vi "Begin.vi"(8 "error in":errorcluster) -> (0 "error out":errorcluster)   [LabVIEW 2017]
doc: "Called before other user functions, this VI is expected to open initial I/O refnums, load in file data, and do all program initialization. Notice that the <B>error out</B> terminal is simply used for data flow. Wiring it to other structures or subVIs ensures that this VI runs first."
uses:
  <vilib>/Rock Robotics/WPI/DriverStation/WPI_DriverStationRobotMode2.ctl
  <vilib>/Rock Robotics/WPI/Joystick/WPI_JoystickDeviceEnum.ctl
  <vilib>/Rock Robotics/WPI/ThirdParty/Phoenix-LabVIEW/Motor Controller/Controls/CTRE_Phoenix_MotorControl_FeedbackDevice.ctl
  <vilib>/Rock Robotics/WPI/ThirdParty/Phoenix-LabVIEW/Motor Controller/Controls/CTRE_Phoenix_MotorControl_NeutralMode.ctl
  <vilib>/Rock Robotics/WPI/ThirdParty/Phoenix-LabVIEW/Motor Controller/Controls/CTRE_Phoenix_MotorControl_ControlMode.ctl
  Robot Global Data.vi
  <vilib>/Rock Robotics/WPI/ThirdParty/Phoenix-LabVIEW/Pigeon IMU/CTRE_PigeonIMU_Open_CAN.vi
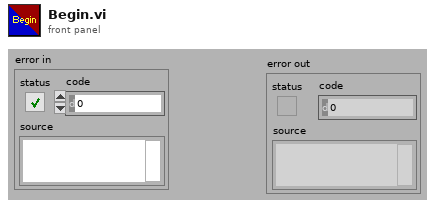
[diagram p1: front panel]
types:
  T1 = typedef "CTRE_Phoenix_MotorControl_ControlMode.ctl" = u16
  T2 = typedef "CTRE_Phoenix_MotorControl_NeutralMode.ctl" = enum8{"EEPROMSetting", "Override to Coast", "Override to Brake"}
  T3 = typedef "CTRE_Phoenix_MotorControl_FeedbackDevice.ctl" = i8
  T4 = typedef "WPI_JoystickDeviceEnum.ctl" = enum16{"USB 0", "USB 1", "USB 2", "USB 3", "USB 4", "USB 5"}
  T5 = typedef "WPI_DriverStationRobotMode2.ctl" = enum16{"Autonomous Disabled", "Autonomous Enabled", "Teleop Disabled", "Teleop Enabled", "Disconnected", "Finish", "Test Disabled", "Test Enabled", "Emergency Stopped"}
  T6 = typedef "CTRE_PigeonIMU_DeviceRef.ctl" = cluster{"DeviceStatus":errorcluster, "Device Number":u8, "Type":T7, "Device ID":u32, "Handle":u64, "UsageFrame":u32, "Library Path":path}
  T7 = typedef "CTRE_PigeonIMU_ConnectionType.ctl" = u32
  T8 = typedef "WPI_JoystickDevRef.ctl" = cluster{"Device":T4}
  T9 = typedef "WPI_MotorControlDeviceRef.ctl" = cluster{"DeviceStatus":errorcluster, "Type":T10, "PWM":cluster{"PWM Channel":T11, "DeadBand":T12}, "CAN":cluster{"Device Number":u8, "SetOutput VI Ref":variant, "GetOutput VI Ref":variant, "Enable VI Ref":variant, "Disable VI Ref":variant, "Data":variant}, "Invert":bool, "DIO PWM":cluster{"PWM \"Enable\" Channel":T11, "DIOChannel":T13, "PWM Rate":dbl}}
  T10 = typedef "WPI_MotorControlType.ctl" = enum16{"PWM", "CAN", "DIO PWM"}
  T11 = typedef "FPGA_DIOPWMChannel.ctl" = enum8{"PWM 0", "PWM 1", "PWM 2", "PWM 3", "PWM 4", "PWM 5", "PWM 6", "PWM 7", "PWM 8", "PWM 9", "PWM MXP 0", "PWM MXP 1", "PWM MXP 2", "PWM MXP 3", "PWM MXP 4", "PWM MXP 5", "PWM MXP 6", "PWM MXP 7", "PWM MXP 8", "PWM MXP 9", "Invalid"}
  T12 = typedef "WPI_PWMDeadband.ctl" = cluster{"Name":string, "maxPositivePwm":i32, "minPositivePwm":i32, "centerPwm":i32, "maxNegativePwm":i32, "minNegativePwm":i32, "angularRange":u16}
  T13 = typedef "FPGA_DIOChannel.ctl" = enum8{"DIO 0", "DIO 1", "DIO 2", "DIO 3", "DIO 4", "DIO 5", "DIO 6", "DIO 7", "DIO 8", "DIO 9", "DIO MXP 0", "DIO MXP 1", "DIO MXP 2", "DIO MXP 3", "DIO MXP 4", "DIO MXP 5", "DIO MXP 6", "DIO MXP 7", "DIO MXP 8", "DIO MXP 9", "DIO MXP 10", "DIO MXP 11", "DIO MXP 12", "DIO MXP 13", "DIO MXP 14", "DIO MXP 15", "SPI Port CS1", "SPI Port CS2", "SPI Port CS3", "SPI Port MISO", "SPI Port MOSI", "Invalid"}
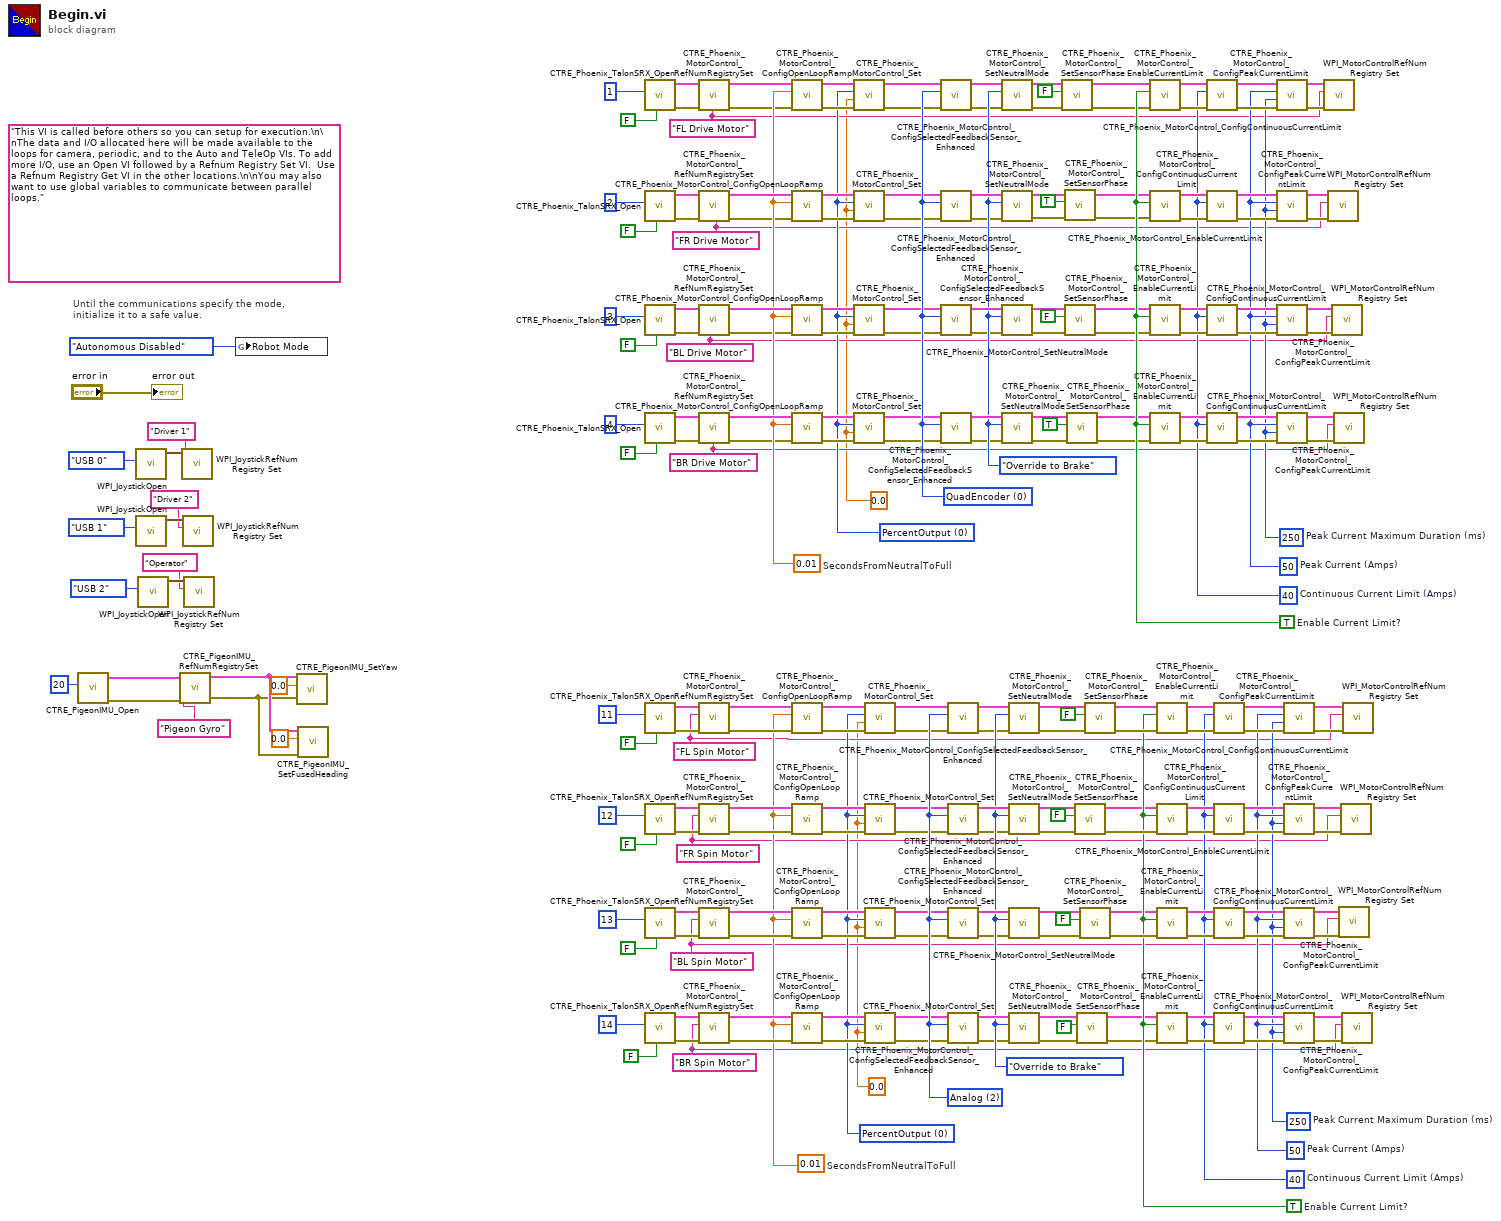
[diagram p0: block diagram]
diagram:
  w1 = 0.0 ("Output")
  w2 = 0.0 ("Output")
  w11 = T1 0 items=["PercentOutput"=0, "Position"=1, "Velocity"=2, "Current"=3, "Follower"=5, "MotionProfile"=6, "MotionMagic"=7, "MotionMagicArc"=8, "MotionProfileArc"=10, "Disabled"=15] ("Control Mode")
  w16 = T1 0 items=["PercentOutput"=0, "Position"=1, "Velocity"=2, "Current"=3, "Follower"=5, "MotionProfile"=6, "MotionMagic"=7, "MotionMagicArc"=8, "MotionProfileArc"=10, "Disabled"=15] ("Control Mode")
  w37 = 0.01  # SecondsFromNeutralToFull
  w94 = CTRE_Phoenix_MotorControl_NeutralMode."Override to Brake" ("Motor Control Neutral Mode")
  w95 = T3 0 items=["None"=-1, "QuadEncoder"=0, "Analog"=2, "Tachometer"=4, "Pulse Width Encoded Position"=8, "Sensor Sum (S0 + S1)"=9, "Sensor Difference (D0 - D1)"=10, "Remote Source 0"=11, "Remote Source 1"=12, "Software Emulated"=15] ("Feedback Device")
  w96 = 0.01  # SecondsFromNeutralToFull
  w7 = "BR Drive Motor" ("refnum name")
  w8 = "BL Drive Motor" ("refnum name")
  w9 = "FR Drive Motor" ("refnum name")
  w62 = 250  # Peak Current Maximum Duration (ms)
  w63 = 50  # Peak Current (Amps)
  w65 = 40  # Continuous Current Limit (Amps)
  w64 = TRUE  # Enable Current Limit?
  w10 = "FL Drive Motor" ("refnum name")
  w173 = CTRE_Phoenix_MotorControl_NeutralMode."Override to Brake" ("Motor Control Neutral Mode")
  w174 = T3 2 items=["None"=-1, "QuadEncoder"=0, "Analog"=2, "Tachometer"=4, "Pulse Width Encoded Position"=8, "Sensor Sum (S0 + S1)"=9, "Sensor Difference (D0 - D1)"=10, "Remote Source 0"=11, "Remote Source 1"=12, "Software Emulated"=15] ("Feedback Device")
  w3 = "BR Spin Motor" ("refnum name")
  w4 = "BL Spin Motor" ("refnum name")
  w5 = "FR Spin Motor" ("refnum name")
  w138 = 250  # Peak Current Maximum Duration (ms)
  w139 = 50  # Peak Current (Amps)
  w141 = 40  # Continuous Current Limit (Amps)
  w140 = TRUE  # Enable Current Limit?
  w6 = "FL Spin Motor" ("refnum name")
  (unwired) "This VI is called before others so you can setup for execution.\n\nThe data and I/O allocated here will be made available to the loops for camera, periodic, and to the Auto and TeleOp VIs. To add more I/O, use an Open VI followed by a Refnum Registry Set VI.  Use a Refnum Registry Get VI in the other locations.\n\nYou may also want to use global variables to communicate between parallel loops."
  # "Until the communications specify the mode,\ninitialize it to a safe value."
  n1 = call-poly <vilib>:"CTRE_PigeonIMU_Open.vi"("Device Number"=u8 20) -> ("error out"=w206:errorcluster, "PigeonIMUDevRef"=w205:T6)  [unwired: 9 in]
  n2 = call <vilib>:"WPI_JoystickOpen.vi"("JoystickDevice"=WPI_JoystickDeviceEnum."USB 0") -> ("JoystickDevRef"=w215:T8)  [unwired: 10 in]
  n3 = call <vilib>:"WPI_JoystickOpen.vi"("JoystickDevice"=WPI_JoystickDeviceEnum."USB 1") -> ("JoystickDevRef"=w214:T8)  [unwired: 10 in]
  n4 = call <vilib>:"WPI_JoystickOpen.vi"("JoystickDevice"=WPI_JoystickDeviceEnum."USB 2") -> ("JoystickDevRef"=w213:T8)  [unwired: 10 in]
  n5 = call <vilib>:"CTRE_PigeonIMU_RefNumRegistrySet.vi"("error in (no error)"=w206, "refnum name"="Pigeon Gyro", "PigeonIMUDevRef"=w205) -> ("error out"=w201:errorcluster, "PigeonIMUDevRef"=w202:T6)  [unwired: 7 in]
  n6 = call <vilib>:"WPI_JoystickRefNum Registry Set.vi"("refnum name"="Driver 1", "JoystickDevRef"=w215) -> ()  [unwired: 8 in, 2 out]
  n7 = call <vilib>:"WPI_JoystickRefNum Registry Set.vi"("refnum name"="Driver 2", "JoystickDevRef"=w214) -> ()  [unwired: 8 in, 2 out]
  n8 = call <vilib>:"WPI_JoystickRefNum Registry Set.vi"("refnum name"="Operator", "JoystickDevRef"=w213) -> ()  [unwired: 8 in, 2 out]
  n9 = global write "Robot Global Data.vi" "Robot Mode"(WPI_DriverStationRobotMode2."Autonomous Disabled" ("Robot Mode")) -> ()
  n10 = call <vilib>:"CTRE_PigeonIMU_SetYaw.vi"("error in (no error)"=w201, "Value"=0.0, "PigeonIMUDevRef"=w202) -> ()  [unwired: 7 in, 2 out]
  n11 = call <vilib>:"CTRE_PigeonIMU_SetFusedHeading.vi"("error in (no error)"=w201, "Value"=0.0, "PigeonIMUDevRef 2"=w202) -> ()  [unwired: 7 in, 2 out]
  n12 = call <vilib>:"CTRE_Phoenix_TalonSRX_Open.vi"("Invert"=FALSE, "Device Number"=u8 1) -> ("error out"=w93:errorcluster, "CAN Talon SRX Ref"=w119:T9)  [unwired: 8 in]
  n13 = call <vilib>:"CTRE_Phoenix_TalonSRX_Open.vi"("Invert"=FALSE, "Device Number"=u8 2) -> ("error out"=w89:errorcluster, "CAN Talon SRX Ref"=w110:T9)  [unwired: 8 in]
  n14 = call <vilib>:"CTRE_Phoenix_TalonSRX_Open.vi"("Invert"=FALSE, "Device Number"=u8 3) -> ("error out"=w85:errorcluster, "CAN Talon SRX Ref"=w105:T9)  [unwired: 8 in]
  n15 = call <vilib>:"CTRE_Phoenix_TalonSRX_Open.vi"("Invert"=FALSE, "Device Number"=u8 4) -> ("error out"=w81:errorcluster, "CAN Talon SRX Ref"=w100:T9)  [unwired: 8 in]
  n16 = call <vilib>:"CTRE_Phoenix_TalonSRX_Open.vi"("Invert"=FALSE, "Device Number"=u8 11) -> ("error out"=w172:errorcluster, "CAN Talon SRX Ref"=w197:T9)  [unwired: 8 in]
  n17 = call <vilib>:"CTRE_Phoenix_TalonSRX_Open.vi"("Invert"=FALSE, "Device Number"=u8 12) -> ("error out"=w168:errorcluster, "CAN Talon SRX Ref"=w188:T9)  [unwired: 8 in]
  n18 = call <vilib>:"CTRE_Phoenix_TalonSRX_Open.vi"("Invert"=FALSE, "Device Number"=u8 13) -> ("error out"=w164:errorcluster, "CAN Talon SRX Ref"=w183:T9)  [unwired: 8 in]
  n19 = call <vilib>:"CTRE_Phoenix_TalonSRX_Open.vi"("Invert"=FALSE, "Device Number"=u8 14) -> ("error out"=w160:errorcluster, "CAN Talon SRX Ref"=w178:T9)  [unwired: 8 in]
  n20 = call <vilib>:"CTRE_Phoenix_MotorControl_RefNumRegistrySet.vi"("error in (no error)"=w93, "refnum name"=w10, "PhoenixMotorControlDevRef"=w119) -> ("error out"=w92:errorcluster, "PhoenixMotorControlDevRef"=w114:T9)  [unwired: 7 in]
  n21 = call <vilib>:"CTRE_Phoenix_MotorControl_RefNumRegistrySet.vi"("error in (no error)"=w89, "refnum name"=w9, "PhoenixMotorControlDevRef"=w110) -> ("error out"=w88:errorcluster, "PhoenixMotorControlDevRef"=w109:T9)  [unwired: 7 in]
  n22 = call <vilib>:"CTRE_Phoenix_MotorControl_RefNumRegistrySet.vi"("error in (no error)"=w85, "refnum name"=w8, "PhoenixMotorControlDevRef"=w105) -> ("error out"=w84:errorcluster, "PhoenixMotorControlDevRef"=w104:T9)  [unwired: 7 in]
  n23 = call <vilib>:"CTRE_Phoenix_MotorControl_RefNumRegistrySet.vi"("error in (no error)"=w81, "refnum name"=w7, "PhoenixMotorControlDevRef"=w100) -> ("error out"=w80:errorcluster, "PhoenixMotorControlDevRef"=w99:T9)  [unwired: 7 in]
  n24 = call <vilib>:"CTRE_Phoenix_MotorControl_RefNumRegistrySet.vi"("error in (no error)"=w172, "refnum name"=w6, "PhoenixMotorControlDevRef"=w197) -> ("error out"=w171:errorcluster, "PhoenixMotorControlDevRef"=w192:T9)  [unwired: 7 in]
  n25 = call <vilib>:"CTRE_Phoenix_MotorControl_RefNumRegistrySet.vi"("error in (no error)"=w168, "refnum name"=w5, "PhoenixMotorControlDevRef"=w188) -> ("error out"=w167:errorcluster, "PhoenixMotorControlDevRef"=w187:T9)  [unwired: 7 in]
  n26 = call <vilib>:"CTRE_Phoenix_MotorControl_RefNumRegistrySet.vi"("error in (no error)"=w164, "refnum name"=w4, "PhoenixMotorControlDevRef"=w183) -> ("error out"=w163:errorcluster, "PhoenixMotorControlDevRef"=w182:T9)  [unwired: 7 in]
  n27 = call <vilib>:"CTRE_Phoenix_MotorControl_RefNumRegistrySet.vi"("error in (no error)"=w160, "refnum name"=w3, "PhoenixMotorControlDevRef"=w178) -> ("error out"=w159:errorcluster, "PhoenixMotorControlDevRef"=w177:T9)  [unwired: 7 in]
  n28 = call <vilib>:"CTRE_Phoenix_MotorControl_ConfigOpenLoopRamp.vi"("error in (no error)"=w92, "secondsFromNeutralToFull"=w96, "PhoenixMotorControlDevRef"=w114) -> ("error out"=w91:errorcluster, "PhoenixMotorControlDevRef"=w113:T9)  [unwired: 7 in]
  n29 = call <vilib>:"CTRE_Phoenix_MotorControl_ConfigOpenLoopRamp.vi"("error in (no error)"=w88, "secondsFromNeutralToFull"=w96, "PhoenixMotorControlDevRef"=w109) -> ("error out"=w87:errorcluster, "PhoenixMotorControlDevRef"=w108:T9)  [unwired: 7 in]
  n30 = call <vilib>:"CTRE_Phoenix_MotorControl_ConfigOpenLoopRamp.vi"("error in (no error)"=w84, "secondsFromNeutralToFull"=w96, "PhoenixMotorControlDevRef"=w104) -> ("error out"=w83:errorcluster, "PhoenixMotorControlDevRef"=w103:T9)  [unwired: 7 in]
  n31 = call <vilib>:"CTRE_Phoenix_MotorControl_ConfigOpenLoopRamp.vi"("error in (no error)"=w80, "secondsFromNeutralToFull"=w96, "PhoenixMotorControlDevRef"=w99) -> ("error out"=w79:errorcluster, "PhoenixMotorControlDevRef"=w98:T9)  [unwired: 7 in]
  n32 = call <vilib>:"CTRE_Phoenix_MotorControl_ConfigOpenLoopRamp.vi"("error in (no error)"=w171, "secondsFromNeutralToFull"=w37, "PhoenixMotorControlDevRef"=w192) -> ("error out"=w170:errorcluster, "PhoenixMotorControlDevRef"=w191:T9)  [unwired: 7 in]
  n33 = call <vilib>:"CTRE_Phoenix_MotorControl_ConfigOpenLoopRamp.vi"("error in (no error)"=w167, "secondsFromNeutralToFull"=w37, "PhoenixMotorControlDevRef"=w187) -> ("error out"=w166:errorcluster, "PhoenixMotorControlDevRef"=w186:T9)  [unwired: 7 in]
  n34 = call <vilib>:"CTRE_Phoenix_MotorControl_ConfigOpenLoopRamp.vi"("error in (no error)"=w163, "secondsFromNeutralToFull"=w37, "PhoenixMotorControlDevRef"=w182) -> ("error out"=w162:errorcluster, "PhoenixMotorControlDevRef"=w181:T9)  [unwired: 7 in]
  n35 = call <vilib>:"CTRE_Phoenix_MotorControl_ConfigOpenLoopRamp.vi"("error in (no error)"=w159, "secondsFromNeutralToFull"=w37, "PhoenixMotorControlDevRef"=w177) -> ("error out"=w158:errorcluster, "PhoenixMotorControlDevRef"=w176:T9)  [unwired: 7 in]
  n36 = call <vilib>:"CTRE_Phoenix_MotorControl_Set.vi"("Output"=w2, "Control Mode"=w11, "PhoenixMotorControlDevRef"=w113) -> ("PhoenixMotorControlDevRef"=w15:T9)  [unwired: 7 in, 1 out]
  n37 = call <vilib>:"CTRE_Phoenix_MotorControl_Set.vi"("Output"=w2, "Control Mode"=w11, "PhoenixMotorControlDevRef"=w108) -> ("PhoenixMotorControlDevRef"=w14:T9)  [unwired: 7 in, 1 out]
  n38 = call <vilib>:"CTRE_Phoenix_MotorControl_Set.vi"("Output"=w2, "Control Mode"=w11, "PhoenixMotorControlDevRef"=w103) -> ("PhoenixMotorControlDevRef"=w13:T9)  [unwired: 7 in, 1 out]
  n39 = call <vilib>:"CTRE_Phoenix_MotorControl_Set.vi"("Output"=w2, "Control Mode"=w11, "PhoenixMotorControlDevRef"=w98) -> ("PhoenixMotorControlDevRef"=w12:T9)  [unwired: 7 in, 1 out]
  n40 = call <vilib>:"CTRE_Phoenix_MotorControl_Set.vi"("Output"=w1, "Control Mode"=w16, "PhoenixMotorControlDevRef"=w191) -> ("PhoenixMotorControlDevRef"=w20:T9)  [unwired: 7 in, 1 out]
  n41 = call <vilib>:"CTRE_Phoenix_MotorControl_Set.vi"("Output"=w1, "Control Mode"=w16, "PhoenixMotorControlDevRef"=w186) -> ("PhoenixMotorControlDevRef"=w19:T9)  [unwired: 7 in, 1 out]
  n42 = call <vilib>:"CTRE_Phoenix_MotorControl_Set.vi"("Output"=w1, "Control Mode"=w16, "PhoenixMotorControlDevRef"=w181) -> ("PhoenixMotorControlDevRef"=w18:T9)  [unwired: 7 in, 1 out]
  n43 = call <vilib>:"CTRE_Phoenix_MotorControl_Set.vi"("Output"=w1, "Control Mode"=w16, "PhoenixMotorControlDevRef"=w176) -> ("PhoenixMotorControlDevRef"=w17:T9)  [unwired: 7 in, 1 out]
  n44 = call <vilib>:"CTRE_Phoenix_MotorControl_ConfigSelectedFeedbackSensor_Enhanced.vi"("error in (no error)"=w91, "Feedback Device"=w95, "PhoenixMotorControlDevRef"=w15) -> ("error out"=w90:errorcluster, "PhoenixMotorControlDevRef"=w112:T9)  [unwired: 7 in]
  n45 = call <vilib>:"CTRE_Phoenix_MotorControl_ConfigSelectedFeedbackSensor_Enhanced.vi"("error in (no error)"=w87, "Feedback Device"=w95, "PhoenixMotorControlDevRef"=w14) -> ("error out"=w86:errorcluster, "PhoenixMotorControlDevRef"=w107:T9)  [unwired: 7 in]
  n46 = call <vilib>:"CTRE_Phoenix_MotorControl_ConfigSelectedFeedbackSensor_Enhanced.vi"("error in (no error)"=w83, "Feedback Device"=w95, "PhoenixMotorControlDevRef"=w13) -> ("error out"=w82:errorcluster, "PhoenixMotorControlDevRef"=w102:T9)  [unwired: 7 in]
  n47 = call <vilib>:"CTRE_Phoenix_MotorControl_ConfigSelectedFeedbackSensor_Enhanced.vi"("error in (no error)"=w79, "Feedback Device"=w95, "PhoenixMotorControlDevRef"=w12) -> ("error out"=w78:errorcluster, "PhoenixMotorControlDevRef"=w97:T9)  [unwired: 7 in]
  n48 = call <vilib>:"CTRE_Phoenix_MotorControl_ConfigSelectedFeedbackSensor_Enhanced.vi"("error in (no error)"=w170, "Feedback Device"=w174, "PhoenixMotorControlDevRef"=w20) -> ("error out"=w169:errorcluster, "PhoenixMotorControlDevRef"=w190:T9)  [unwired: 7 in]
  n49 = call <vilib>:"CTRE_Phoenix_MotorControl_ConfigSelectedFeedbackSensor_Enhanced.vi"("error in (no error)"=w166, "Feedback Device"=w174, "PhoenixMotorControlDevRef"=w19) -> ("error out"=w165:errorcluster, "PhoenixMotorControlDevRef"=w185:T9)  [unwired: 7 in]
  n50 = call <vilib>:"CTRE_Phoenix_MotorControl_ConfigSelectedFeedbackSensor_Enhanced.vi"("error in (no error)"=w162, "Feedback Device"=w174, "PhoenixMotorControlDevRef"=w18) -> ("error out"=w161:errorcluster, "PhoenixMotorControlDevRef"=w180:T9)  [unwired: 7 in]
  n51 = call <vilib>:"CTRE_Phoenix_MotorControl_ConfigSelectedFeedbackSensor_Enhanced.vi"("error in (no error)"=w158, "Feedback Device"=w174, "PhoenixMotorControlDevRef"=w17) -> ("error out"=w157:errorcluster, "PhoenixMotorControlDevRef"=w175:T9)  [unwired: 7 in]
  n52 = call <vilib>:"CTRE_Phoenix_MotorControl_SetNeutralMode.vi"("error in (no error)"=w90, "Motor Control Neutral Mode"=w94, "PhoenixMotorControlDevRef"=w112) -> ("error out"=w51:errorcluster, "PhoenixMotorControlDevRef"=w52:T9)  [unwired: 7 in]
  n53 = call <vilib>:"CTRE_Phoenix_MotorControl_SetNeutralMode.vi"("error in (no error)"=w86, "Motor Control Neutral Mode"=w94, "PhoenixMotorControlDevRef"=w107) -> ("error out"=w47:errorcluster, "PhoenixMotorControlDevRef"=w48:T9)  [unwired: 7 in]
  n54 = call <vilib>:"CTRE_Phoenix_MotorControl_SetNeutralMode.vi"("error in (no error)"=w82, "Motor Control Neutral Mode"=w94, "PhoenixMotorControlDevRef"=w102) -> ("error out"=w41:errorcluster, "PhoenixMotorControlDevRef"=w42:T9)  [unwired: 7 in]
  n55 = call <vilib>:"CTRE_Phoenix_MotorControl_SetNeutralMode.vi"("error in (no error)"=w78, "Motor Control Neutral Mode"=w94, "PhoenixMotorControlDevRef"=w97) -> ("error out"=w56:errorcluster, "PhoenixMotorControlDevRef"=w57:T9)  [unwired: 7 in]
  n56 = call <vilib>:"CTRE_Phoenix_MotorControl_SetNeutralMode.vi"("error in (no error)"=w169, "Motor Control Neutral Mode"=w173, "PhoenixMotorControlDevRef"=w190) -> ("error out"=w152:errorcluster, "PhoenixMotorControlDevRef"=w133:T9)  [unwired: 7 in]
  n57 = call <vilib>:"CTRE_Phoenix_MotorControl_SetNeutralMode.vi"("error in (no error)"=w165, "Motor Control Neutral Mode"=w173, "PhoenixMotorControlDevRef"=w185) -> ("error out"=w149:errorcluster, "PhoenixMotorControlDevRef"=w132:T9)  [unwired: 7 in]
  n58 = call <vilib>:"CTRE_Phoenix_MotorControl_SetNeutralMode.vi"("error in (no error)"=w161, "Motor Control Neutral Mode"=w173, "PhoenixMotorControlDevRef"=w180) -> ("error out"=w146:errorcluster, "PhoenixMotorControlDevRef"=w131:T9)  [unwired: 7 in]
  n59 = call <vilib>:"CTRE_Phoenix_MotorControl_SetNeutralMode.vi"("error in (no error)"=w157, "Motor Control Neutral Mode"=w173, "PhoenixMotorControlDevRef"=w175) -> ("error out"=w129:errorcluster, "PhoenixMotorControlDevRef"=w130:T9)  [unwired: 7 in]
  n60 = call <vilib>:"CTRE_Phoenix_MotorControl_SetSensorPhase.vi"("error in (no error)"=w51, "PhaseSensor"=FALSE, "PhoenixMotorControlDevRef"=w52) -> ("error out"=w49:errorcluster, "PhoenixMotorControlDevRef"=w50:T9)  [unwired: 7 in]
  n61 = call <vilib>:"CTRE_Phoenix_MotorControl_SetSensorPhase.vi"("error in (no error)"=w47, "PhaseSensor"=TRUE, "PhoenixMotorControlDevRef"=w48) -> ("error out"=w46:errorcluster, "PhoenixMotorControlDevRef"=w45:T9)  [unwired: 7 in]
  n62 = call <vilib>:"CTRE_Phoenix_MotorControl_SetSensorPhase.vi"("error in (no error)"=w41, "PhaseSensor"=FALSE, "PhoenixMotorControlDevRef"=w42) -> ("error out"=w40:errorcluster, "PhoenixMotorControlDevRef"=w39:T9)  [unwired: 7 in]
  n63 = call <vilib>:"CTRE_Phoenix_MotorControl_SetSensorPhase.vi"("error in (no error)"=w56, "PhaseSensor"=TRUE ("Invert?"), "PhoenixMotorControlDevRef"=w57) -> ("error out"=w54:errorcluster, "PhoenixMotorControlDevRef"=w53:T9)  [unwired: 7 in]
  n64 = call <vilib>:"CTRE_Phoenix_MotorControl_SetSensorPhase.vi"("PhaseSensor"=FALSE, "PhoenixMotorControlDevRef"=w132) -> ("PhoenixMotorControlDevRef"=w124:T9)  [unwired: 8 in, 1 out]
  n65 = call <vilib>:"CTRE_Phoenix_MotorControl_SetSensorPhase.vi"("PhaseSensor"=FALSE, "PhoenixMotorControlDevRef"=w130) -> ("PhoenixMotorControlDevRef"=w128:T9)  [unwired: 8 in, 1 out]
  n66 = call <vilib>:"CTRE_Phoenix_MotorControl_SetSensorPhase.vi"("PhaseSensor"=FALSE, "PhoenixMotorControlDevRef"=w131) -> ("PhoenixMotorControlDevRef"=w126:T9)  [unwired: 8 in, 1 out]
  n67 = call <vilib>:"CTRE_Phoenix_MotorControl_SetSensorPhase.vi"("PhaseSensor"=FALSE, "PhoenixMotorControlDevRef"=w133) -> ("PhoenixMotorControlDevRef"=w122:T9)  [unwired: 8 in, 1 out]
  n68 = call <vilib>:"CTRE_Phoenix_MotorControl_EnableCurrentLimit.vi"("error in (no error)"=w49, "Enable Current Limit?"=w64, "PhoenixMotorControlDevRef"=w50) -> ("error out"=w73:errorcluster, "PhoenixMotorControlDevRef"=w75:T9)  [unwired: 7 in]
  n69 = call <vilib>:"CTRE_Phoenix_MotorControl_EnableCurrentLimit.vi"("error in (no error)"=w46, "Enable Current Limit?"=w64, "PhoenixMotorControlDevRef"=w45) -> ("error out"=w71:errorcluster, "PhoenixMotorControlDevRef"=w77:T9)  [unwired: 7 in]
  n70 = call <vilib>:"CTRE_Phoenix_MotorControl_EnableCurrentLimit.vi"("error in (no error)"=w40, "Enable Current Limit?"=w64, "PhoenixMotorControlDevRef"=w39) -> ("error out"=w69:errorcluster, "PhoenixMotorControlDevRef"=w118:T9)  [unwired: 7 in]
  n71 = call <vilib>:"CTRE_Phoenix_MotorControl_EnableCurrentLimit.vi"("error in (no error)"=w54, "Enable Current Limit?"=w64, "PhoenixMotorControlDevRef"=w53) -> ("error out"=w67:errorcluster, "PhoenixMotorControlDevRef"=w116:T9)  [unwired: 7 in]
  n72 = call <vilib>:"CTRE_Phoenix_MotorControl_EnableCurrentLimit.vi"("error in (no error)"=w152, "Enable Current Limit?"=w140, "PhoenixMotorControlDevRef"=w122) -> ("error out"=w151:errorcluster, "PhoenixMotorControlDevRef"=w154:T9)  [unwired: 7 in]
  n73 = call <vilib>:"CTRE_Phoenix_MotorControl_EnableCurrentLimit.vi"("error in (no error)"=w149, "Enable Current Limit?"=w140, "PhoenixMotorControlDevRef"=w124) -> ("error out"=w148:errorcluster, "PhoenixMotorControlDevRef"=w156:T9)  [unwired: 7 in]
  n74 = call <vilib>:"CTRE_Phoenix_MotorControl_EnableCurrentLimit.vi"("error in (no error)"=w146, "Enable Current Limit?"=w140, "PhoenixMotorControlDevRef"=w126) -> ("error out"=w145:errorcluster, "PhoenixMotorControlDevRef"=w196:T9)  [unwired: 7 in]
  n75 = call <vilib>:"CTRE_Phoenix_MotorControl_EnableCurrentLimit.vi"("error in (no error)"=w129, "Enable Current Limit?"=w140, "PhoenixMotorControlDevRef"=w128) -> ("error out"=w143:errorcluster, "PhoenixMotorControlDevRef"=w194:T9)  [unwired: 7 in]
  n76 = call <vilib>:"CTRE_Phoenix_MotorControl_ConfigContinuousCurrentLimit.vi"("error in (no error)"=w73, "Continuous Current Limit (Amps)"=w65, "PhoenixMotorControlDevRef"=w75) -> ("error out"=w72:errorcluster, "PhoenixMotorControlDevRef"=w74:T9)  [unwired: 7 in]
  n77 = call <vilib>:"CTRE_Phoenix_MotorControl_ConfigContinuousCurrentLimit.vi"("error in (no error)"=w71, "Continuous Current Limit (Amps)"=w65, "PhoenixMotorControlDevRef"=w77) -> ("error out"=w70:errorcluster, "PhoenixMotorControlDevRef"=w76:T9)  [unwired: 7 in]
  n78 = call <vilib>:"CTRE_Phoenix_MotorControl_ConfigContinuousCurrentLimit.vi"("error in (no error)"=w69, "Continuous Current Limit (Amps)"=w65, "PhoenixMotorControlDevRef"=w118) -> ("error out"=w68:errorcluster, "PhoenixMotorControlDevRef"=w117:T9)  [unwired: 7 in]
  n79 = call <vilib>:"CTRE_Phoenix_MotorControl_ConfigContinuousCurrentLimit.vi"("error in (no error)"=w67, "Continuous Current Limit (Amps)"=w65, "PhoenixMotorControlDevRef"=w116) -> ("error out"=w66:errorcluster, "PhoenixMotorControlDevRef"=w115:T9)  [unwired: 7 in]
  n80 = call <vilib>:"CTRE_Phoenix_MotorControl_ConfigContinuousCurrentLimit.vi"("error in (no error)"=w151, "Continuous Current Limit (Amps)"=w141, "PhoenixMotorControlDevRef"=w154) -> ("error out"=w150:errorcluster, "PhoenixMotorControlDevRef"=w153:T9)  [unwired: 7 in]
  n81 = call <vilib>:"CTRE_Phoenix_MotorControl_ConfigContinuousCurrentLimit.vi"("error in (no error)"=w148, "Continuous Current Limit (Amps)"=w141, "PhoenixMotorControlDevRef"=w156) -> ("error out"=w147:errorcluster, "PhoenixMotorControlDevRef"=w155:T9)  [unwired: 7 in]
  n82 = call <vilib>:"CTRE_Phoenix_MotorControl_ConfigContinuousCurrentLimit.vi"("error in (no error)"=w145, "Continuous Current Limit (Amps)"=w141, "PhoenixMotorControlDevRef"=w196) -> ("error out"=w144:errorcluster, "PhoenixMotorControlDevRef"=w195:T9)  [unwired: 7 in]
  n83 = call <vilib>:"CTRE_Phoenix_MotorControl_ConfigContinuousCurrentLimit.vi"("error in (no error)"=w143, "Continuous Current Limit (Amps)"=w141, "PhoenixMotorControlDevRef"=w194) -> ("error out"=w142:errorcluster, "PhoenixMotorControlDevRef"=w193:T9)  [unwired: 7 in]
  n84 = call <vilib>:"CTRE_Phoenix_MotorControl_ConfigPeakCurrentLimit.vi"("error in (no error)"=w72, "Peak Current Maximum Duration (ms)"=w62, "Peak Current (Amps)"=w63, "PhoenixMotorControlDevRef"=w74) -> ("error out"=w36:errorcluster, "PhoenixMotorControlDevRef"=w35:T9)  [unwired: 6 in]
  n85 = call <vilib>:"CTRE_Phoenix_MotorControl_ConfigPeakCurrentLimit.vi"("error in (no error)"=w70, "Peak Current Maximum Duration (ms)"=w62, "Peak Current (Amps)"=w63, "PhoenixMotorControlDevRef"=w76) -> ("error out"=w34:errorcluster, "PhoenixMotorControlDevRef"=w33:T9)  [unwired: 6 in]
  n86 = call <vilib>:"CTRE_Phoenix_MotorControl_ConfigPeakCurrentLimit.vi"("error in (no error)"=w68, "Peak Current Maximum Duration (ms)"=w62, "Peak Current (Amps)"=w63, "PhoenixMotorControlDevRef"=w117) -> ("error out"=w32:errorcluster, "PhoenixMotorControlDevRef"=w31:T9)  [unwired: 6 in]
  n87 = call <vilib>:"CTRE_Phoenix_MotorControl_ConfigPeakCurrentLimit.vi"("error in (no error)"=w66, "Peak Current Maximum Duration (ms)"=w62, "Peak Current (Amps)"=w63, "PhoenixMotorControlDevRef"=w115) -> ("error out"=w30:errorcluster, "PhoenixMotorControlDevRef"=w29:T9)  [unwired: 6 in]
  n88 = call <vilib>:"CTRE_Phoenix_MotorControl_ConfigPeakCurrentLimit.vi"("error in (no error)"=w150, "Peak Current Maximum Duration (ms)"=w138, "Peak Current (Amps)"=w139, "PhoenixMotorControlDevRef"=w153) -> ("error out"=w28:errorcluster, "PhoenixMotorControlDevRef"=w27:T9)  [unwired: 6 in]
  n89 = call <vilib>:"CTRE_Phoenix_MotorControl_ConfigPeakCurrentLimit.vi"("error in (no error)"=w147, "Peak Current Maximum Duration (ms)"=w138, "Peak Current (Amps)"=w139, "PhoenixMotorControlDevRef"=w155) -> ("error out"=w26:errorcluster, "PhoenixMotorControlDevRef"=w25:T9)  [unwired: 6 in]
  n90 = call <vilib>:"CTRE_Phoenix_MotorControl_ConfigPeakCurrentLimit.vi"("error in (no error)"=w144, "Peak Current Maximum Duration (ms)"=w138, "Peak Current (Amps)"=w139, "PhoenixMotorControlDevRef"=w195) -> ("error out"=w24:errorcluster, "PhoenixMotorControlDevRef"=w23:T9)  [unwired: 6 in]
  n91 = call <vilib>:"CTRE_Phoenix_MotorControl_ConfigPeakCurrentLimit.vi"("error in (no error)"=w142, "Peak Current Maximum Duration (ms)"=w138, "Peak Current (Amps)"=w139, "PhoenixMotorControlDevRef"=w193) -> ("error out"=w22:errorcluster, "PhoenixMotorControlDevRef"=w21:T9)  [unwired: 6 in]
  n92 = call <vilib>:"WPI_MotorControlRefNum Registry Set.vi"("error in (no error)"=w36, "refnum name"=w10, "MotorControlDevRef"=w35) -> ()  [unwired: 7 in, 2 out]
  n93 = call <vilib>:"WPI_MotorControlRefNum Registry Set.vi"("error in (no error)"=w34, "refnum name"=w9, "MotorControlDevRef"=w33) -> ()  [unwired: 7 in, 2 out]
  n94 = call <vilib>:"WPI_MotorControlRefNum Registry Set.vi"("error in (no error)"=w32, "refnum name"=w8, "MotorControlDevRef"=w31) -> ()  [unwired: 7 in, 2 out]
  n95 = call <vilib>:"WPI_MotorControlRefNum Registry Set.vi"("error in (no error)"=w30, "refnum name"=w7, "MotorControlDevRef"=w29) -> ()  [unwired: 7 in, 2 out]
  n96 = call <vilib>:"WPI_MotorControlRefNum Registry Set.vi"("error in (no error)"=w24, "refnum name"=w4, "MotorControlDevRef"=w23) -> ()  [unwired: 7 in, 2 out]
  n97 = call <vilib>:"WPI_MotorControlRefNum Registry Set.vi"("error in (no error)"=w26, "refnum name"=w5, "MotorControlDevRef"=w25) -> ()  [unwired: 7 in, 2 out]
  n98 = call <vilib>:"WPI_MotorControlRefNum Registry Set.vi"("error in (no error)"=w22, "refnum name"=w3, "MotorControlDevRef"=w21) -> ()  [unwired: 7 in, 2 out]
  n99 = call <vilib>:"WPI_MotorControlRefNum Registry Set.vi"("error in (no error)"=w28, "refnum name"=w6, "MotorControlDevRef"=w27) -> ()  [unwired: 7 in, 2 out]
  "error out" <- "error in"
